vi "MouseChirp-Create.vi"(11 "error in (no error)":errorcluster, 12 "Fs (Hz)":dbl) -> (8 "Array":dbl[](array[numeric]), 15 "error out":errorcluster)   [LabVIEW 2015]
uses:
  Utility VIs/Math VIs/LinSpace (x0-dx-npts).vi
  Utility VIs/Math VIs/FFT x(t) to dB,Degrees (1D).vi
panel:
  out "XY Graph":T1(graph)
  in  "Ramp (ms)":dbl=0.1
  in  "Fmax (Hz)":dbl=60000.0
  in  "Fmin (Hz)":dbl=4000.0
  in  "Sweep Rate (Hz/s)":dbl=42900000.0
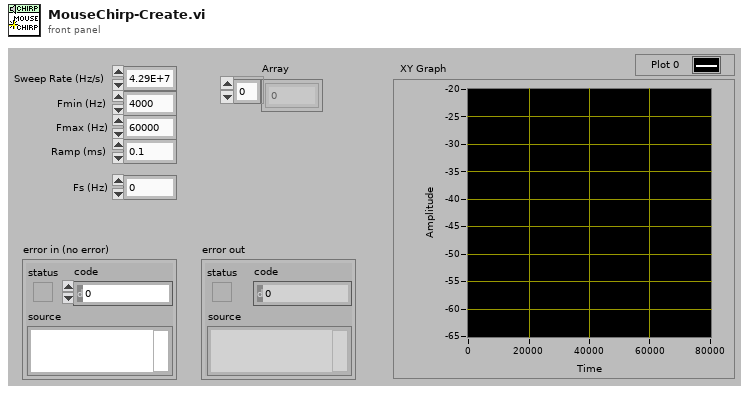
[diagram p1: front panel]
types:
  T1 = cluster{"+Freq. Mag of FFT (dB rms)":dbl[], "Array":dbl[]}
  T2 = cluster{"Active":bool, "Delay (ms)":dbl, "Width (ms)":dbl, "Ramp (ms)":dbl}
  T3 = cluster{"Array":dbl[], "+Freq. Mag of FFT (dB rms)":dbl[]}
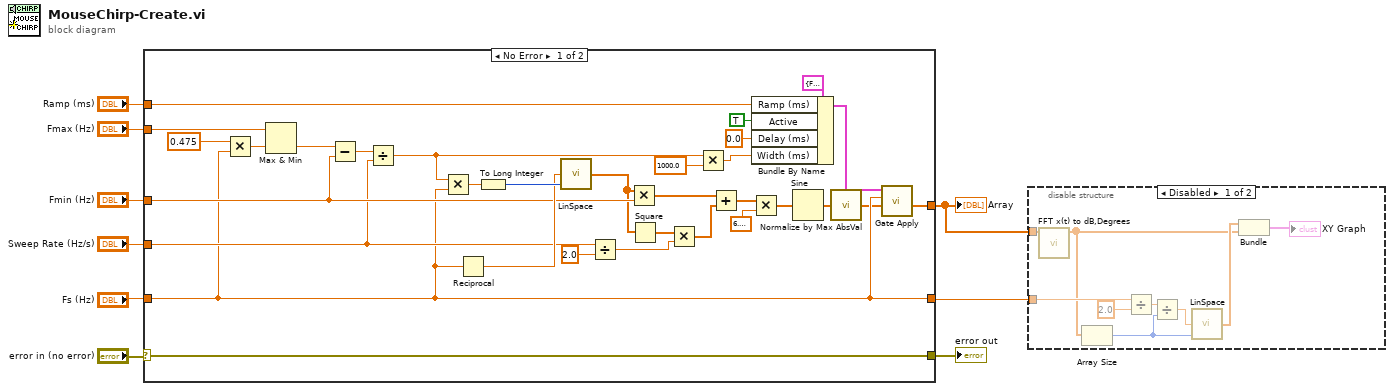
[diagram p0: block diagram]
diagram:
  n1 = case shown="No Error" "error in (no error)" {
    selector: "error in (no error)" -> [w41 w42]
    tunnel: [w41 w42] -> w8
    tunnel: "Fmax (Hz)" -> [w40 _]
    tunnel: "Fs (Hz)" -> [w11 _]
    tunnel: "Fmin (Hz)" -> [w32 _]
    tunnel: "Sweep Rate (Hz/s)" -> [w31 _]
    tunnel: [w19 _] -> w2
    tunnel: "Ramp (ms)" -> [w14 _]
    tunnel: [w11 _] -> w1
    frame No Error {
      n2 = Multiply(x=0.475 ("y"), y=w11) -> (x*y=w39:dbl)
      n3 = Max & Min(x=w40, y=w39) -> (min(x,y)=w37:dbl)  [unwired: 1 out]
      n4 = Subtract(x=w37, y=w32) -> (x-y=w36:dbl)
      n5 = Divide(x=w36, y=w31) -> (x/y=w15:dbl)
      n6 = Multiply(x=w15, y=w11) -> (x*y=w35:dbl)
      n7 = Reciprocal(x=w11) -> (1/x=w33:dbl)
      n8 = To Long Integer(number=w35) -> (32bit integer=w34:i32)
      n9 = call-poly "LinSpace.vi"("npts"=w34, "dx"=w33) -> ("Array"=w29:dbl[])  [unwired: 2 in, 1 out]
      n10 = Divide(x=w31, y=2.0) -> (x/y=w27:dbl)
      n11 = Multiply(x=w29, y=w32) -> (x*y=w26:dbl[])
      n12 = Square(x=w29) -> (x^2=w28:dbl[])
      n13 = Multiply(x=w28, y=w27) -> (x*y=w25:dbl[])
      n14 = Multiply(x=w15, y=1000.0) -> (x*y=w13:dbl)
      n15 = Add(x=w26, y=w25) -> (x+y=w24:dbl[])
      n16 = Multiply(x=w24, y=6.283185307179586) -> (x*y=w22:dbl[])
      n17 = Bundle By Name(cluster=T2 {"Active"=FALSE, "Delay (ms)"=0.0, "Width (ms)"=0.0, "Ramp (ms)"=0.0} ("Gate Control"), "Ramp (ms)"=w14, "Active"=TRUE, "Delay (ms)"=0.0, "Width (ms)"=w13) -> (w18:T2)
      n18 = Sine(x=w22) -> (sin(x)=w21:dbl[])
      n19 = call "Normalize by Max AbsVal.vi"("Y"=w21) -> ("Ynorm"=w10:dbl[])
      n20 = call "Gate Apply.vi"("Waveform in"=w10, "Sampling Rate (Hz)"=w11, "Gate Control"=w18) -> ("Gated waveform"=w19:dbl[])  [unwired: 7 in, 1 out]
    }
    frame Error {
    }
  }
  "error out" <- w8
  "Array" <- w2
  n21 = disable-structure shown="Disabled" {
    disable-tunnel: w2 -> [w51 _]
    disable-tunnel: w1 -> [w49 _]
    frame Disabled {
      n22 = call-poly "FFT x(t) to dB,Degrees.vi"("X"=w51) -> ("+Freq. Mag of FFT (dB rms)"=w43:dbl[])  [unwired: 8 in, 2 out]
      n23 = Array Size(array=w43) -> (size(s)=w46:i32)
      n24 = Divide(x=w49, y=2.0) -> (x/y=w47:dbl)
      n25 = Divide(x=w47, y=w46) -> (x/y=w45:dbl)
      n26 = call-poly "LinSpace.vi"("npts"=w46, "dx"=w45) -> ("Array"=w44:dbl[])  [unwired: 2 in, 1 out]
      n27 = Bundle("Array"=w44, "+Freq. Mag of FFT (dB rms)"=w43) -> (→"XY Graph":T3)  [unwired: 1 in]
    }
    frame Enabled {
    }
  }
